vi "Method.vi"(4 "Value":refnum<class "Abs_Time.lvclass">) -> (1 "Result":refnum<class "Abs_Time.lvclass">)   [LabVIEW 2021, in "Increment_Time.lvclass"]
uses:
  Increment_Time.lvclass
  Abs_Types/Time/Abs_Time.lvclass
  C:/TSA/LV_Abstract/Source/Functions/Support/Function/One Terminal/Time/AbsFunc_One Term_Time.lvclass
  C:/Program Files (x86)/National Instruments/LabVIEW 2021/vi.lib/TSA/Abstract Data Classes/Abs_Types/Time/Abs_Time.lvclass
  Support/Function/One Terminal/Time/AbsFunc_One Term_Time.lvclass/AbsFunc_One Term_Time.ctl
  Support/Function/One Terminal/Time/Properties/Write Numeric A.vi
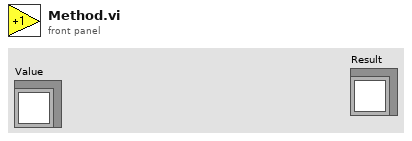
[diagram p1: front panel]
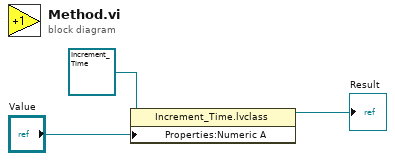
[diagram p0: block diagram]
diagram:
  n1 = property class="Increment_Time.lvclass"(reference=refnum<class "Increment_Time.lvclass"> refnum ("Decrement_DBL.lvclass"), "Properties:Numeric A"="Value") -> (reference out=→"Result":refnum<class "Increment_Time.lvclass">)  [unwired: 1 in, 1 out]
